vi "ADIS16470 Process Example.vi"(8 "error in (no error)":errorcluster, 11 "element":T1) -> (0 "error out":errorcluster)   [LabVIEW 2018]
uses:
  Typedef/ADIS16470 Data.ctl
  <vilib>/ptbypt/NI_PtbyPt.lvlib
panel:
  out "Average Time Delta":dbl
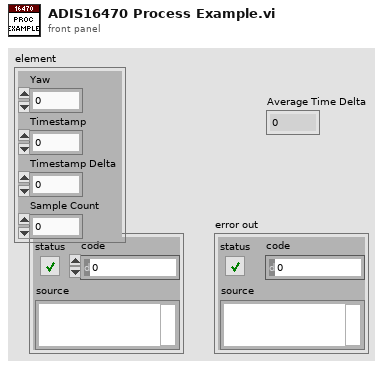
[diagram p1: front panel]
types:
  T1 = typedef "ADIS16470 Data.ctl" = cluster{"Yaw":dbl, "Timestamp":dbl, "Timestamp Delta":dbl, "Sample Count":u16}
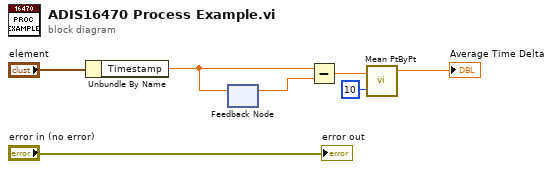
[diagram p0: block diagram]
diagram:
  n1 = Unbundle By Name("element") -> ("Timestamp"=w5:dbl)
  n2 = feedback-in #1(w5) -> ()
  n3 = feedback #1() -> (w4:dbl)  [unwired: 1 in]
  n4 = Subtract(x=w5, y=w4) -> (x-y=w3:dbl)
  n5 = call <vilib>:"Mean PtByPt.vi"("x"=w3, "sample length"=10) -> ("mean"=→"Average Time Delta":dbl)  [unwired: 2 in, 1 out]
  "error out" <- "error in (no error)"
